vi "String_Convert_Upper_Lower.vi"() -> ()   [LabVIEW 2019]
panel:
  out "all upper case string":string
  out "all lower case string 2":string
  out "all lower case string":string
  in  "String 4":string
  in  "String 2":string
  in  "String":string
  # "String Upper Lower"
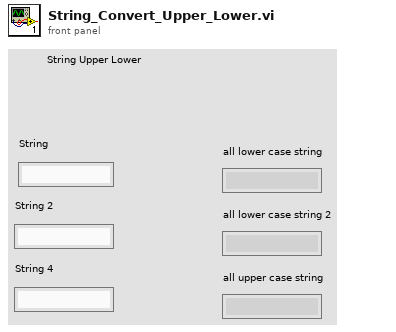
[diagram p1: front panel]
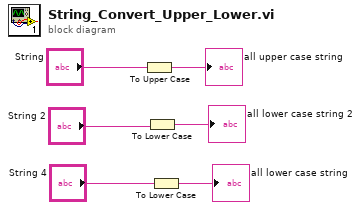
[diagram p0: block diagram]
diagram:
  n1 = To Upper Case(1:"String") -> (0:→"all upper case string":string)
  n2 = To Lower Case(string="String 2") -> (all lower case string=→"all lower case string 2":string)
  n3 = To Lower Case(string="String 4") -> (all lower case string=→"all lower case string":string)
